vi "ConnectedStatus.vi"(8 "error in (no error)":errorcluster, 11 "ChromaAcLoad in":refnum<class "ChromaAcLoad.lvclass">) -> (0 "error out":errorcluster, 2 "Any Connections?":bool, 3 "ChromaAcLoad out":refnum<class "ChromaAcLoad.lvclass">)   [LabVIEW 2018, in "AcPwrPlugins.lvlib" / "ChromaAcLoad.lvclass"]
doc: "This VI displays the boolean status of if the instrumetn is connected i.e. a valid reference to the instrument has been established."
uses:
  ChromaAcLoad.lvclass
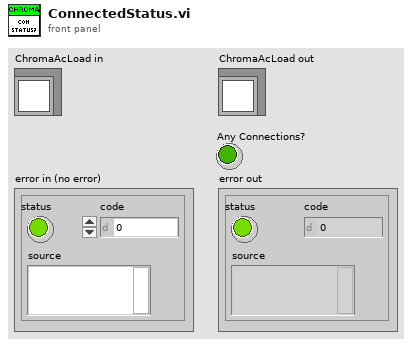
[diagram p1: front panel]
types:
  T1 = cluster{"Handle":string, "Name":string, "Phase Select":i32, "Instrument Options":string, "id query (T)":bool, "reset device (T)":bool, "Load Short Circuited":bool, "Line Synchronization":bool, "Load Current (A/Arms)":dbl, "Load Voltage (V/Vrms)":dbl, "Load Power (W)":dbl, "Load Resistance (Ohms)":dbl, "Load Current Peak Limit (A)":dbl, "Load Current Limit (A/Arms)":dbl, "Load Power Limit (W)":dbl, "Synch Frequency (Hz)":dbl, "Priority":enum16{"CF Only", "PF Only", "Both (CF)", "Both (PF)"}, "Crest Factor":dbl, "Power Factor":dbl, "Slew Rate":cluster{"Rise Slew Rate (A/ms)":i32, "Fall Slew Rate (A/ms)":i32}, "LC/RLC Mode":cluster{"Capacitance (uF)":i32, "Inductance (uH)":i32, "Series Resistance (Ohm)":dbl, "Parallel Resistance (Ohm)":dbl}, "Timing":cluster{"TimingOn":enum16{""}, "Hours":u32, "Minutes":u32, "Seconds":dbl, "CutoffVoltage":dbl}, "Connected":bool}[]
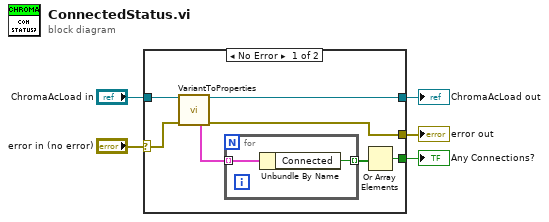
[diagram p0: block diagram]
diagram:
  n1 = case shown="No Error" "error in (no error)" {
    selector: "error in (no error)" -> [w10 w15]
    tunnel: "ChromaAcLoad in" -> [w9 w16]
    tunnel: [w7 w16] -> w3
    tunnel: [w8 w15] -> w2
    tunnel: [w12 _] -> w1
    frame No Error {
      n2 = call "VariantToProperties.vi"("ChromaAcLoad"=w9, "error in (no error)"=w10) -> ("ChromaAcLoad"=w7:refnum<class "ChromaAcLoad.lvclass">, "Phases"=w6:T1, "error out"=w8:errorcluster)  [unwired: 7 in, 4 out]
      n3 = for {
        tunnel: w6 -> [w14] mode=indexing
        tunnel: [w13] -> w11 mode=indexing
        n4 = Unbundle By Name(w14) -> ("Connected"=w13:bool)
      }
      n5 = Or Array Elements(Boolean array=w11) -> (logical OR=w12:bool)
    }
    frame Error {
    }
  }
  "ChromaAcLoad out" <- w3
  "error out" <- w2
  "Any Connections?" <- w1
